vi "simplegrab.vi"() -> ()   [LabVIEW 2010]
panel:
  out "Picture Out":picture
  in  "ICImagingControl":refnum<k7>(container)
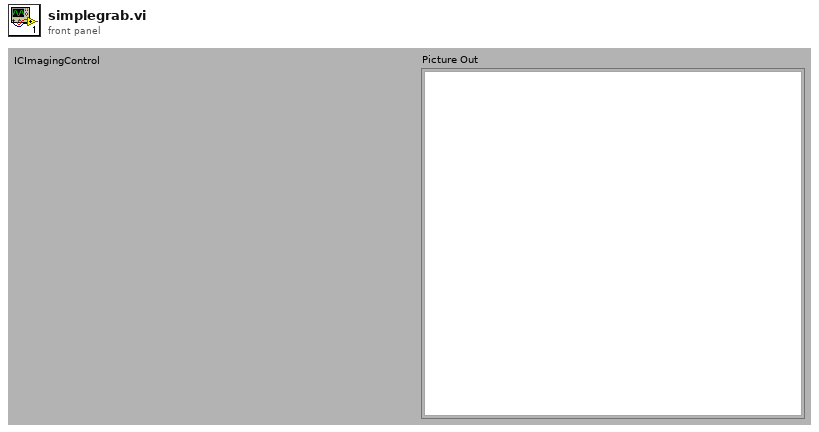
[diagram p1: front panel]
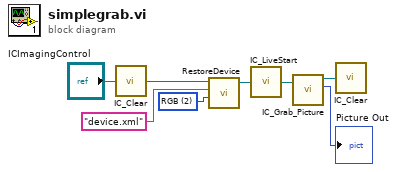
[diagram p0: block diagram]
diagram:
  w6 = u16 2 items=["RGB"=2, "Y800"=5, "Y16"=11] ("Color modes")
  n1 = call <userlib>:"IC_Clear.vi"("ICImagingControl 2"="ICImagingControl") -> ("ICImagingControl"=w7:refnum<k7>)
  n2 = call <userlib>:"RestoreDevice.vi"("Color modes"=w6, "Filename"="device.xml", "ICImagingControl"=w7) -> ("ICImagingControl 2"=w5:refnum<k7>)  [unwired: 1 in, 2 out]
  n3 = call <userlib>:"IC_LiveStart.vi"("ICImagingControl 3"=w5) -> ("ICImagingControl 2"=w4:refnum<k7>)
  n4 = call <userlib>:"IC_Grab_Picture.vi"("ICImagingControl In"=w4) -> ("ICImagingControl Out"=w3:refnum<k7>, "Picture Out"=→"Picture Out":picture)  [unwired: 1 in, 2 out]
  n5 = call <userlib>:"IC_Clear.vi"("ICImagingControl 2"=w3) -> ()  [unwired: 1 out]
